vi "current-instance.vi"() -> ()   [LabVIEW 2016, in "test-find-vi-by-name.lvlib"]
uses:
  test-find-vi-by-name.lvlib
  <vilib>/addons/_JKI Toolkits/Caraya/classes/Assert/Assert Equal Value_Variant.vi
  <vilib>/addons/_JKI Toolkits/Caraya/classes/Test/Test.lvclass
  <vilib>/addons/_JKI Toolkits/Caraya/classes/Assert/Assert.lvclass
  main/apis/Application/Application.lvclass
panel:
  out "error out":errorcluster
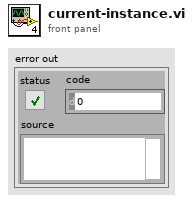
[diagram p1: front panel]
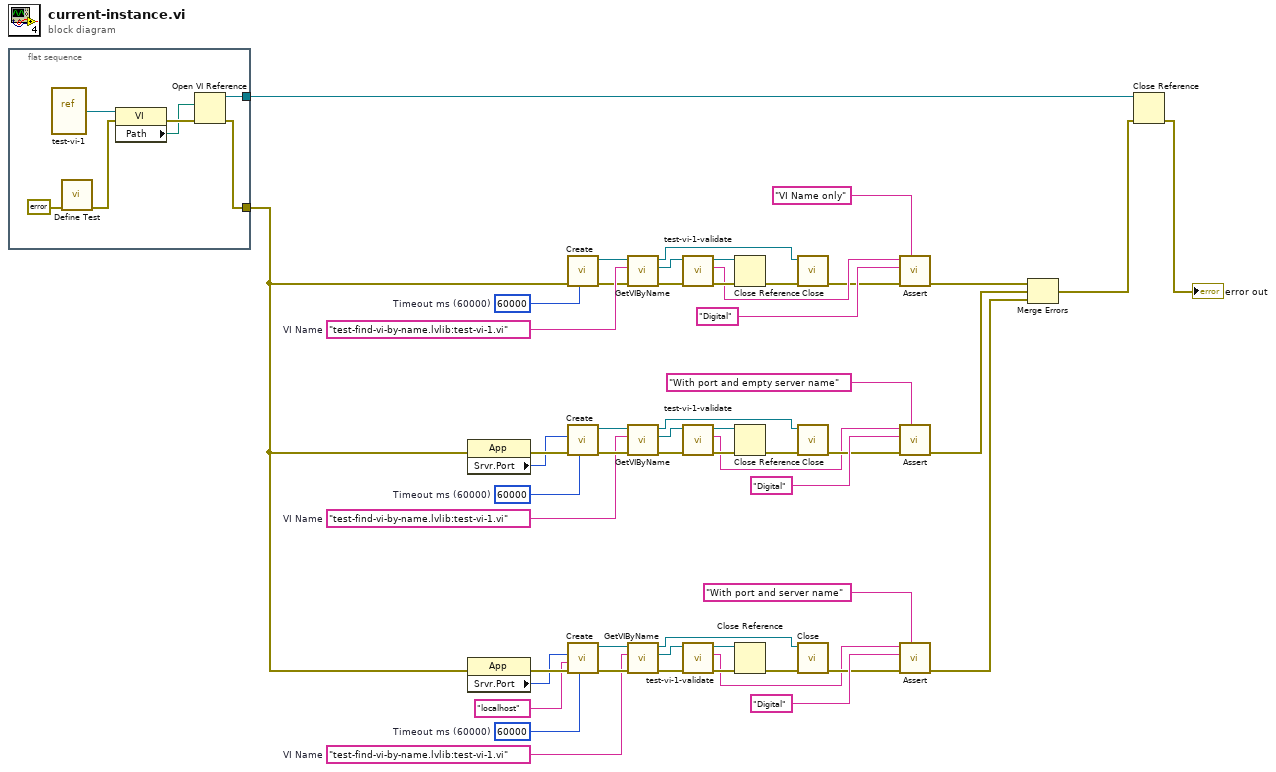
[diagram p0: block diagram]
diagram:
  w2 = 60000  # Timeout ms (60000)
  w5 = "test-find-vi-by-name.lvlib:test-vi-1.vi"  # VI Name
  w17 = 60000  # Timeout ms (60000)
  w16 = "test-find-vi-by-name.lvlib:test-vi-1.vi"  # VI Name
  w40 = 60000  # Timeout ms (60000)
  w38 = "test-find-vi-by-name.lvlib:test-vi-1.vi"  # VI Name
  n1 = flat-sequence {
    tunnel: [w57] -> w34
    tunnel: [w56] -> w41
    frame #0 {
      n2 = vi-ref "test-vi-1.vi"() -> (w59:refnum<vi>)
      n3 = call <vilib>:"Define Test.vi"("error in (no error)"=errorcluster {"status"=FALSE, "code"=0, "source"=""}) -> ("error out"=w60:errorcluster)  [unwired: 10 in]
      n4 = property on="Property Node" class="VI"(reference=w59, error in=w60) -> (error out=w58:errorcluster, "Path"=w55:path)  [unwired: 1 out]
      n5 = Open VI Reference(vi path=w55, error in (no error)=w58) -> (vi reference=w56:refnum<vi>, error out=w57:errorcluster)  [unwired: 4 in]
    }
  }
  n6 = property on="Property Node" class="App"(error in=w34) -> (error out=w21:errorcluster, "Srvr.Port"=w18:u32)  [unwired: 1 in, 1 out]
  n7 = property on="Property Node" class="App"(error in=w34) -> (error out=w7:errorcluster, "Srvr.Port"=w4:u32)  [unwired: 1 in, 1 out]
  n8 = call "Create.vi"("Timeout ms (60000)"=w40, "error in (no error)"=w34) -> ("error out"=w33:errorcluster, "Application out"=w37:refnum<class "Application.lvclass">)  [unwired: 8 in]
  n9 = call "Create.vi"("Timeout ms (60000)"=w17, "error in (no error)"=w21, "Port(0:Ignored)"=w18) -> ("error out"=w28:errorcluster, "Application out"=w25:refnum<class "Application.lvclass">)  [unwired: 7 in]
  n10 = call "Create.vi"("Timeout ms (60000)"=w2, "error in (no error)"=w7, "Service Name (\"\":localhost)"="localhost" ("Service Name (\"\":localhost)"), "Port(0:Ignored)"=w4) -> ("error out"=w9:errorcluster, "Application out"=w12:refnum<class "Application.lvclass">)  [unwired: 6 in]
  n11 = call "GetVIByName.vi"("error in (no error)"=w33, "VI Name"=w38, "Application in"=w37) -> ("error out"=w39:errorcluster, "VI Reference"=w35:refnum<vi>, "Application out"=w36:refnum<class "Application.lvclass">)  [unwired: 6 in]
  n12 = call "GetVIByName.vi"("error in (no error)"=w28, "VI Name"=w16, "Application in"=w25) -> ("error out"=w24:errorcluster, "VI Reference"=w27:refnum<vi>, "Application out"=w26:refnum<class "Application.lvclass">)  [unwired: 6 in]
  n13 = call "GetVIByName.vi"("error in (no error)"=w9, "VI Name"=w5, "Application in"=w12) -> ("error out"=w13:errorcluster, "VI Reference"=w10:refnum<vi>, "Application out"=w11:refnum<class "Application.lvclass">)  [unwired: 6 in]
  n14 = call "test-vi-1-validate.vi"("error in (no error)"=w39, "VI in"=w35) -> ("error out"=w52:errorcluster, "ClassName"=w50:string, "VI out"=w51:refnum<vi>)  [unwired: 7 in]
  n15 = call "test-vi-1-validate.vi"("error in (no error)"=w24, "VI in"=w27) -> ("error out"=w22:errorcluster, "ClassName"=w19:string, "VI out"=w23:refnum<vi>)  [unwired: 7 in]
  n16 = call "test-vi-1-validate.vi"("error in (no error)"=w13, "VI in"=w10) -> ("error out"=w15:errorcluster, "ClassName"=w1:string, "VI out"=w14:refnum<vi>)  [unwired: 7 in]
  n17 = Close Reference(reference=w51, error in (no error)=w52) -> (error out=w31:errorcluster)
  n18 = Close Reference(reference=w23, error in (no error)=w22) -> (error out=w29:errorcluster)
  n19 = Close Reference(reference=w14, error in (no error)=w15) -> (error out=w8:errorcluster)
  n20 = call "Close.vi"("error in (no error)"=w31, "Application in"=w36) -> ("error out"=w30:errorcluster)  [unwired: 9 in]
  n21 = call "Close.vi"("error in (no error)"=w29, "Application in"=w26) -> ("error out"=w20:errorcluster)  [unwired: 9 in]
  n22 = call "Close.vi"("error in (no error)"=w8, "Application in"=w11) -> ("error out"=w6:errorcluster)  [unwired: 9 in]
  n23 = call-poly <vilib>:"Assert.vi"("Label"="VI Name only" ("Label (VI Title)"), "error in (no error)"=w30, "Y"="Digital" ("Class Name"), "X"=w50) -> ("error out"=w53:errorcluster)  [unwired: 7 in]
  n24 = call-poly <vilib>:"Assert.vi"("Label"="With port and empty server name" ("Label (VI Title)"), "error in (no error)"=w20, "Y"="Digital" ("Class Name"), "X"=w19) -> ("error out"=w46:errorcluster)  [unwired: 7 in]
  n25 = call-poly <vilib>:"Assert.vi"("Label"="With port and server name" ("Label (VI Title)"), "error in (no error)"=w6, "Y"="Digital" ("Class Name"), "X"=w1) -> ("error out"=w43:errorcluster)  [unwired: 7 in]
  n26 = Merge Errors(w53, w46, w43) -> (w32:errorcluster)
  n27 = Close Reference(reference=w41, error in (no error)=w32) -> (error out=→"error out":errorcluster)
